vi "Viewer.vi"() -> ()   [LabVIEW 2015]
uses:
  <vilib>/addons/database/Auxilliary.llb/DB Tools DataTypes.ctl
  <vilib>/addons/database/Connection.llb/DB Tools Open Connec (Path).vi
  <vilib>/addons/database/NI_Database_API.lvlib
panel:
  out "columns":string[][](array[string])
  out "column information":T2(array[cluster])
  out "tables":string[](array[string])
  in  "connection information":path
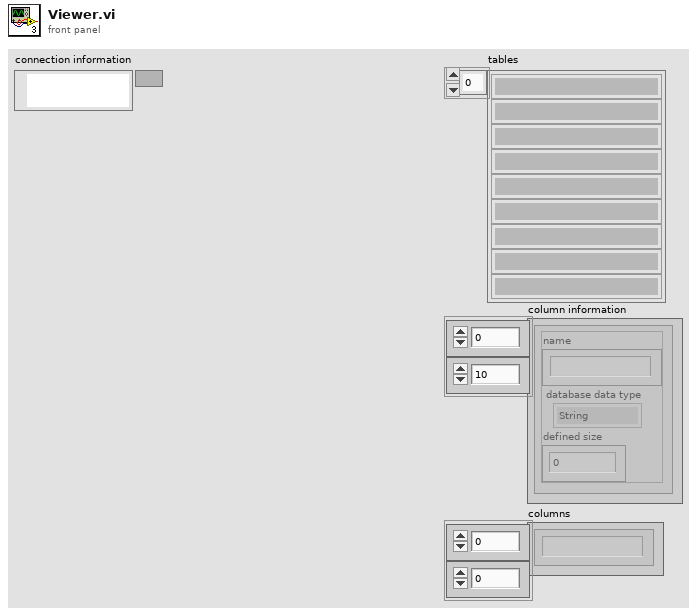
[diagram p1: front panel]
types:
  T1 = typedef "NI_Database_API.lvlib/DB Tools DataTypes.ctl" = enum16{"String", "Long (I32)", "Single (SGL)", "Double (DBL)", "Date/Time", "Binary"}
  T2 = cluster{"name":string, "database data type":T1, "defined size":i32}[][]
  T3 = typedef "NI_Database_API.lvlib/Conn ObjectReference.ctl" = refnum<k1>
  T4 = cluster{"name":string, "database data type":T1, "defined size":i32}[]
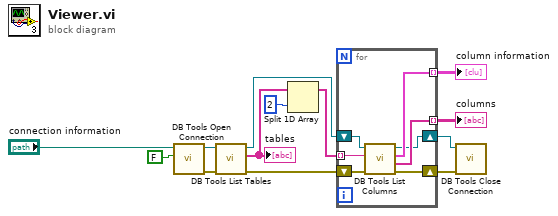
[diagram p0: block diagram]
diagram:
  n1 = call-poly <vilib>:"DB Tools Open Connection.vi"("prompt? (F)"=FALSE, "connection information"="connection information") -> ("error out"=w10:errorcluster, "connection reference"=w11:T3)  [unwired: 6 in]
  n2 = call <vilib>:"DB Tools List Tables.vi"("error in (no error)"=w10, "connection reference"=w11) -> ("error out"=w7:errorcluster, "tables"=w8:string[], "connection reference out"=w9:T3)  [unwired: 3 in]
  "tables" <- w8
  n3 = Split 1D Array(array=w8, index=2) -> (first subarray=w2:string[])  [unwired: 1 out]
  n4 = for {
    shift-right: [w16] -> w6
    shift-left: w9 -> [w17]
    tunnel: w2 -> [w20] mode=indexing
    tunnel: [w19] -> w4 mode=indexing
    tunnel: [w18] -> w3 mode=indexing
    shift-right: [w14] -> w5
    shift-left: w7 -> [w15]
    n5 = call <vilib>:"DB Tools List Columns.vi"("error in (no error)"=w15, "table"=w20, "connection reference"=w17) -> ("error out"=w14:errorcluster, "columns"=w18:string[], "column information"=w19:T4, "connection reference out"=w16:T3)  [unwired: 1 in]
  }
  "column information" <- w4
  "columns" <- w3
  n6 = call <vilib>:"DB Tools Close Connection.vi"("error in (no error)"=w5, "connection reference"=w6) -> ()  [unwired: 5 in, 1 out]
